vi "Untitled 1.vi"() -> ()   [LabVIEW 2012]
uses:
  TV/RW/Includes/WLAN - TV - OPPO - RW - INC - TV_Rx_Measurements.ctl
  TV/RW/Includes/WLAN - NIStandardDefine.ctl
panel:
  out "error out":errorcluster
  in  "Rx Measurements Settings":T1={"Channel Bandwidth (Hz)"=4.0, "Idle Interval (s)"=40000000.0, "MCS Index"=0, "80211n PLCP Frame Format"=0, "Payload Data Length (bytes)"=0, "OFDM Data Rate (Mbps)"=1024, "DSSS Data Rate (Mbps)"=0, "#N_SS"=0, "NIStandard"=enum."80211A/G/J/P(OFDM)"} {"DSSS Data Rate (Mbps)" items=["1", "2", "5.5 CCK", "5.5 PBCC", "11 CCK", "11 PBCC", "22", "33"]; "OFDM Data Rate (Mbps)" items=["6", "9", "12", "18", "24", "36", "48", "54"]; "80211n PLCP Frame Format" items=["Mixed Format", "Greenfield Format"]}
  in  "RFSG Handle":string
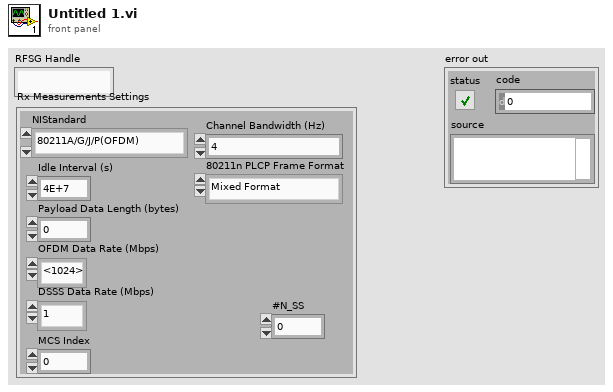
[diagram p1: front panel]
types:
  T1 = typedef "WLAN - TV - OPPO - RW - INC - TV_Rx_Measurements.ctl" = cluster{"Channel Bandwidth (Hz)":dbl, "Idle Interval (s)":dbl, "MCS Index":i32, "80211n PLCP Frame Format":i32, "Payload Data Length (bytes)":i32, "OFDM Data Rate (Mbps)":i32, "DSSS Data Rate (Mbps)":i32, "#N_SS":i32, "NIStandard":T2}
  T2 = typedef "WLAN - NIStandardDefine.ctl" = enum32{"80211A/G/J/P(OFDM)", "80211B/G(DSSS)", "80211GDSSSOFDM", "80211NMIMOOFDM", "80211ACMIMOOFDM"}
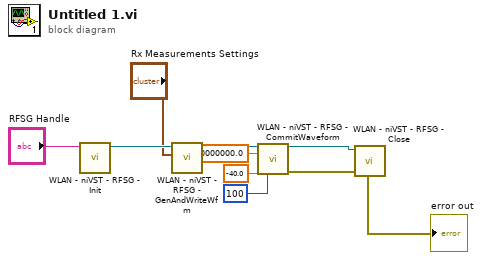
[diagram p0: block diagram]
diagram:
  n1 = call "WLAN - niVST - RFSG - Init.vi"("RFSG Handle"="RFSG Handle") -> ("RFSG handle out"=w9:refnum<k15>)  [unwired: 9 in, 1 out]
  n2 = call "WLAN - niVST - RFSG - GenAndWriteWfm.vi"("Rx Measurements Settings"="Rx Measurements Settings", "instrument handle"=w9) -> ("RFSG out"=w8:refnum<k15>)  [unwired: 8 in, 1 out]
  n3 = call "WLAN - niVST - RFSG - CommitWaveform.vi"("RFSG handle"=w8, "RF:Frequency (Hz)"=5180000000.0, "RxPower"=-40.0, "Number of Packets"=100) -> ("RFSG handle out"=w7:refnum<k15>, "error out"=→"error out":errorcluster)  [unwired: 10 in]
  n4 = call "WLAN - niVST - RFSG - Close.vi"("RFSG handle"=w7) -> ()  [unwired: 10 in, 1 out]
